vi "Write Page General Properties.vi"(8 "Error In":errorcluster, 10 "General Page Properties":T1, 11 "Custom Device Page .NET Ref In":refnum<k24>) -> (0 "Error Out":errorcluster, 3 "Custom Device Page .NET Ref Out":refnum<k24>)   [LabVIEW 2019, in "VeriStand Custom Device XML Parser.lvlib"]
doc: "Sets the general properties of a custom device page"
uses:
  VeriStand Custom Device XML Parser.lvlib
  NationalInstruments.VeriStand.XMLReader
  XML Controls/Page Properties.ctl
  XML Controls/Path Cluster.ctl
  XML Controls/Help File Properties.ctl
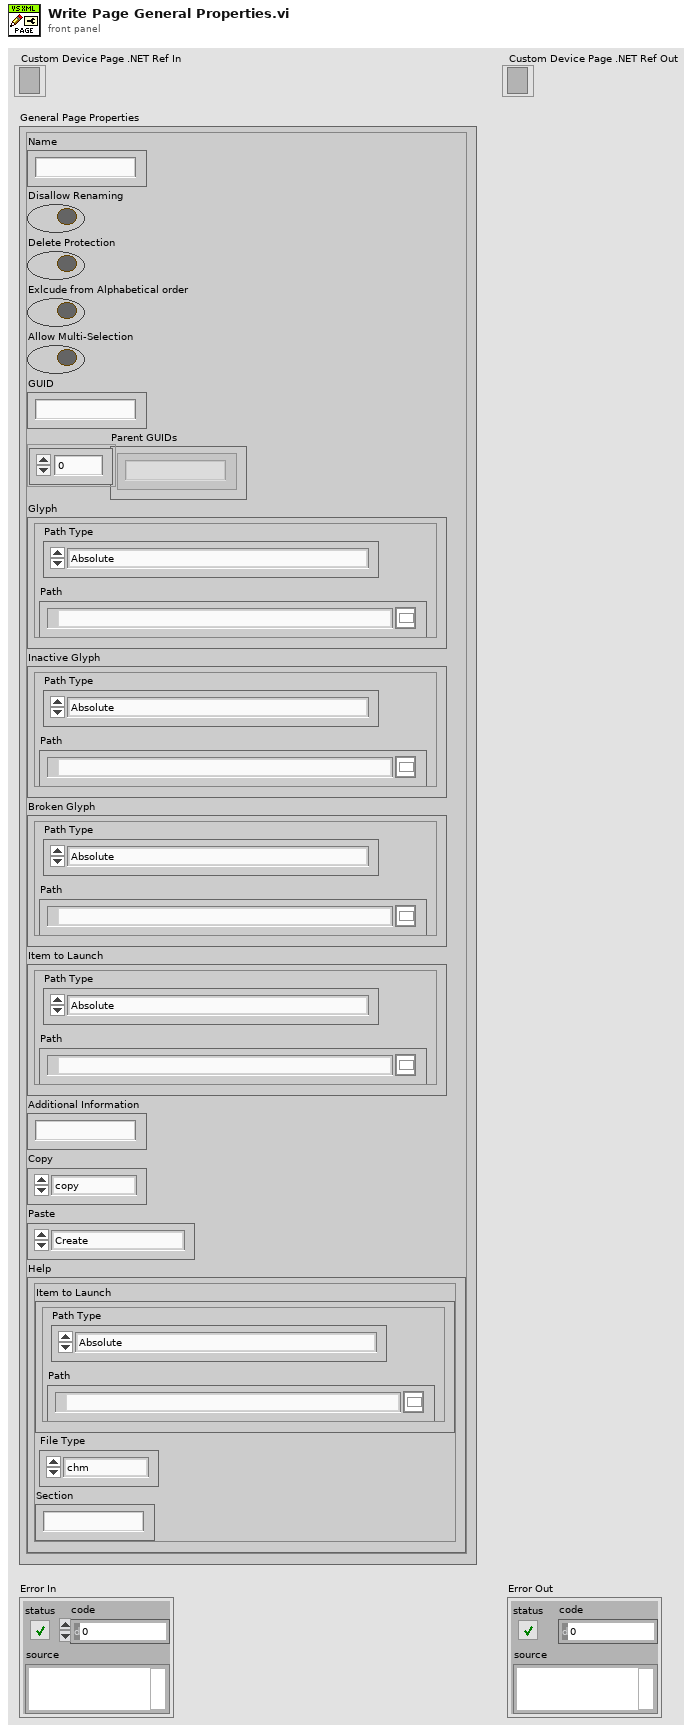
[diagram p1: front panel]
types:
  T1 = typedef "VeriStand Custom Device XML Parser.lvlib/Page Properties.ctl" = cluster{"Name":string, "Disallow Renaming":bool, "Delete Protection":bool, "Exlcude from Alphabetical order":bool, "Allow Multi-Selection":bool, "GUID":string, "Parent GUIDs":string[], "Glyph":T2, "Inactive Glyph":T2, "Broken Glyph":T2, "Item to Launch":T2, "Additional Information":string, "Copy":enum16{"copy", "disabled"}, "Paste":enum16{"Create", "CreatIfNotExists_GUID", "CreatIfNotExists_Name", "Replace", "Dialog"}, "Help":T3}
  T2 = typedef "VeriStand Custom Device XML Parser.lvlib/Path Cluster.ctl" = cluster{"Path":path, "Path Type":enum16{"Absolute", "To Base", "To Common Doc Dir", "To Application Data Dir"}}
  T3 = typedef "VeriStand Custom Device XML Parser.lvlib/Help File Properties.ctl" = cluster{"Item to Launch":T2, "Section":string, "File Type":enum16{"chm", "other"}}
  T4 = enum16{"Create", "CreatIfNotExists_GUID", "CreatIfNotExists_Name", "Replace", "Dialog"}
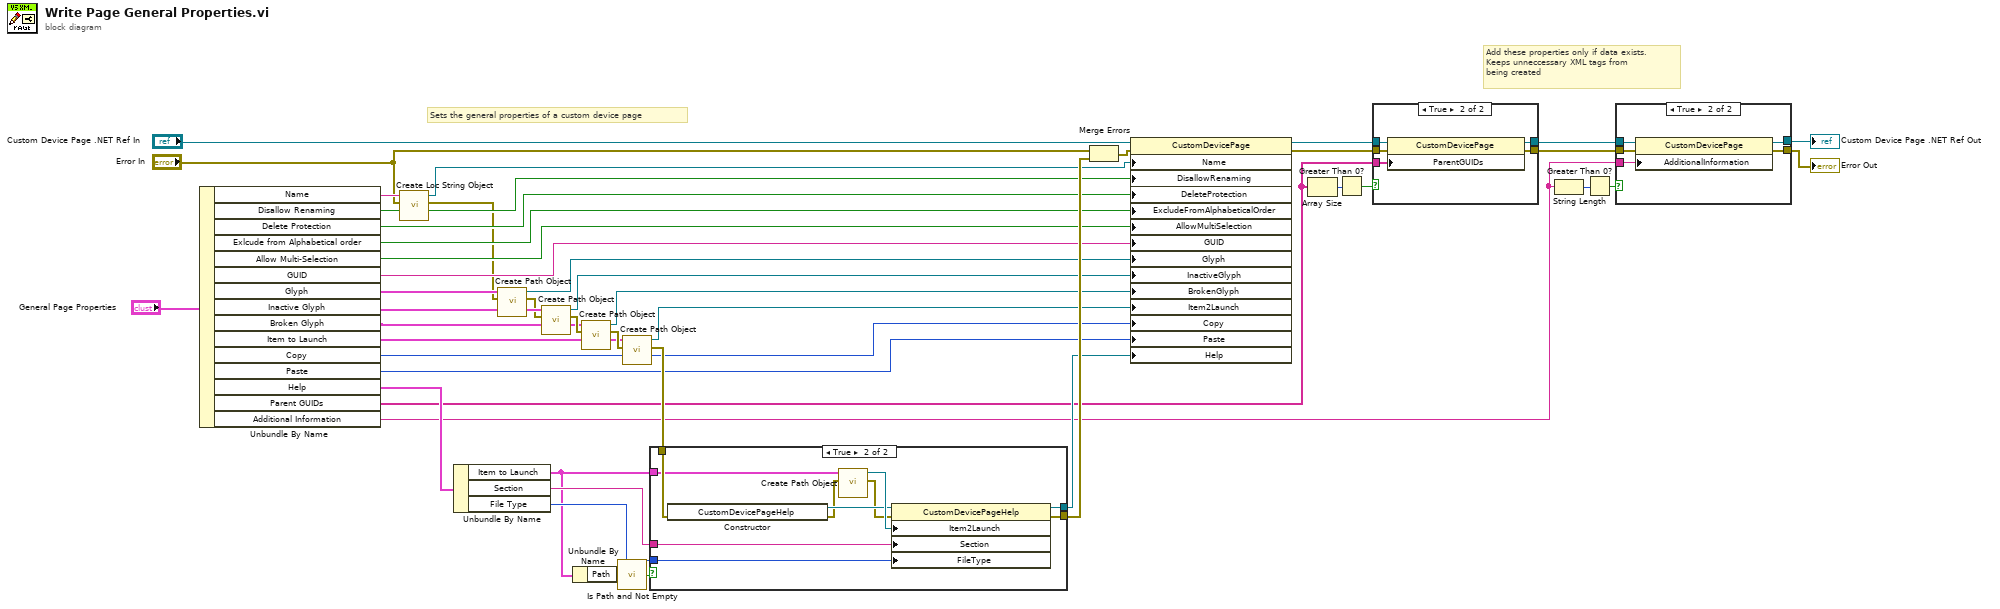
[diagram p0: block diagram]
diagram:
  # "Add these properties only if data exists.\nKeeps unneccessary XML tags from\nbeing created"
  # "Sets the general properties of a custom device page"
  n1 = Unbundle By Name("General Page Properties") -> ("Name"=w20:string, "Disallow Renaming"=w22:bool, "Delete Protection"=w23:bool, "Exlcude from Alphabetical order"=w24:bool, "Allow Multi-Selection"=w25:bool, "GUID"=w26:string, "Glyph"=w27:T2, "Inactive Glyph"=w30:T2, "Broken Glyph"=w32:T2, "Item to Launch"=w35:T2, "Copy"=w38:enum16{"copy", "disabled"}, "Paste"=w39:T4, "Help"=w40:T3, "Parent GUIDs"=w8:string[], "Additional Information"=w3:string)
  n2 = call "Create Loc String Object.vi"("Error In"="Error In", "String Input"=w20) -> ("Error Out"=w16:errorcluster, "Loc String .NET Ref"=w21:refnum<k24>)  [unwired: 8 in]
  n3 = Unbundle By Name(w40) -> ("Item to Launch"=w15:T2, "Section"=w42:string, "File Type"=w43:enum16{"chm", "other"})
  n4 = call "Create Path Object.vi"("Error In"=w16, "Path Data Cluster"=w27) -> ("Error Out"=w29:errorcluster, "Path .NET Ref"=w28:refnum<k24>)  [unwired: 8 in]
  n5 = call "Create Path Object.vi"("Error In"=w29, "Path Data Cluster"=w30) -> ("Error Out"=w33:errorcluster, "Path .NET Ref"=w31:refnum<k24>)  [unwired: 8 in]
  n6 = Unbundle By Name(w15) -> ("Path"=w14:path)
  n7 = call "Create Path Object.vi"("Error In"=w33, "Path Data Cluster"=w32) -> ("Error Out"=w36:errorcluster, "Path .NET Ref"=w34:refnum<k24>)  [unwired: 8 in]
  n8 = call <vilib>:"Is Path and Not Empty.vi"("path"=w14) -> ("Is Path and Not Empty?"=w13:bool)  [unwired: 4 in]
  n9 = call "Create Path Object.vi"("Error In"=w36, "Path Data Cluster"=w35) -> ("Error Out"=w41:errorcluster, "Path .NET Ref"=w37:refnum<k24>)  [unwired: 8 in]
  n10 = case shown="True" w13 {
    tunnel: [w47 w57] -> w46
    tunnel: [_ w56] -> w44
    tunnel: w43 -> [_ w55]
    tunnel: w42 -> [_ w54]
    tunnel: w41 -> [w47 w49]
    tunnel: w15 -> [_ w48]
    frame False {
    }
    frame True {
      n11 = constructor class="CustomDevicePageHelp"(error in=w49) -> (reference out=w52:refnum<k24>, error out=w50:errorcluster)  [unwired: 2 in, 1 out]
      n12 = call "Create Path Object.vi"("Error In"=w50, "Path Data Cluster"=w48) -> ("Error Out"=w51:errorcluster, "Path .NET Ref"=w53:refnum<k24>)  [unwired: 8 in]
      n13 = property class="CustomDevicePageHelp"(reference=w52, error in=w51, "Item2Launch"=w53, "Section"=w54, "FileType"=w55) -> (reference out=w56:refnum<k24>, error out=w57:errorcluster)
    }
  }
  n14 = Merge Errors("Error In", w46) -> (w45:errorcluster)
  n15 = property class="CustomDevicePage"(reference="Custom Device Page .NET Ref In", error in=w45, "Name"=w21, "DisallowRenaming"=w22, "DeleteProtection"=w23, "ExcludeFromAlphabeticalOrder"=w24, "AllowMultiSelection"=w25, "GUID"=w26, "Glyph"=w28, "InactiveGlyph"=w31, "BrokenGlyph"=w34, "Item2Launch"=w37, "Copy"=w38, "Paste"=w39, "Help"=w44) -> (reference out=w12:refnum<k24>, error out=w11:errorcluster)
  n16 = Array Size(array=w8) -> (size(s)=w7:i32)
  n17 = Greater Than 0?(x=w7) -> (x > 0?=w6:bool)
  n18 = case shown="True" w6 {
    tunnel: w12 -> [w59 w64]
    tunnel: w11 -> [w58 w63]
    tunnel: [w59 w62] -> w10
    tunnel: [w58 w61] -> w9
    tunnel: w8 -> [_ w60]
    frame False {
    }
    frame True {
      n19 = property class="CustomDevicePage"(reference=w64, error in=w63, "ParentGUIDs"=w60) -> (reference out=w62:refnum<k24>, error out=w61:errorcluster)
    }
  }
  n20 = String Length(string=w3) -> (length=w5:i32)
  n21 = Greater Than 0?(x=w5) -> (x > 0?=w4:bool)
  n22 = case shown="True" w4 {
    tunnel: w10 -> [w66 w71]
    tunnel: w9 -> [w65 w70]
    tunnel: [w66 w69] -> w2
    tunnel: [w65 w68] -> w1
    tunnel: w3 -> [_ w67]
    frame False {
    }
    frame True {
      n23 = property class="CustomDevicePage"(reference=w71, error in=w70, "AdditionalInformation"=w67) -> (reference out=w69:refnum<k24>, error out=w68:errorcluster)
    }
  }
  "Error Out" <- w1
  "Custom Device Page .NET Ref Out" <- w2
